vi "generateWaveform.vi"(8 "error in (no error)":errorcluster, 11 "GuassianNoiseWave in":refnum<class "GuassianNoiseWave.lvclass">) -> (0 "error out":errorcluster, 2 "signal out":waveform(dbl), 3 "GuassianNoiseWave out":refnum<class "GuassianNoiseWave.lvclass">)   [LabVIEW 2015, in "GuassianNoiseWave.lvclass"]
uses:
  GuassianNoiseWave.lvclass
  GuassianNoiseWave.lvclass/GuassianNoiseWave.ctl
  <vilib>/Waveform/WDTOps.llb/WDT Append Waveforms DBL.vi
  <vilib>/measure/NI_MABase.lvlib
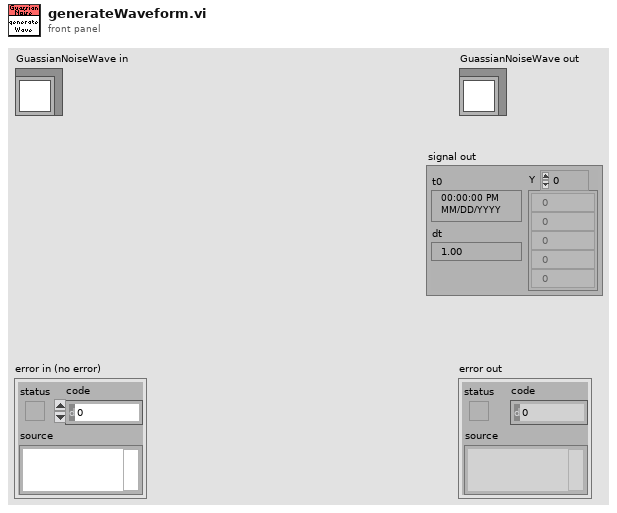
[diagram p1: front panel]
types:
  T1 = typedef "FAMTTypedefs.lvlib/Iterations.ctl" = i32
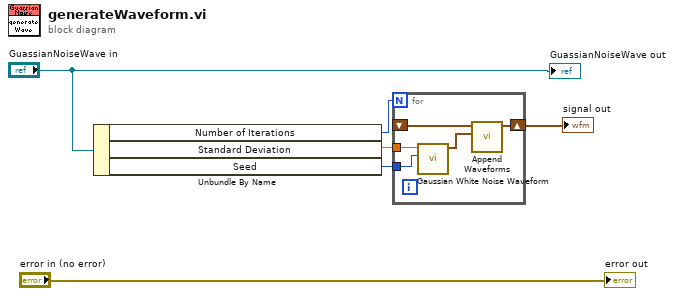
[diagram p0: block diagram]
diagram:
  n1 = Unbundle By Name("GuassianNoiseWave in") -> ("Number of Iterations"=w4:T1, "Standard Deviation"=w6:dbl, "Seed"=w5:i32)
  n2 = for {
    N: w4 -> [_]
    tunnel: w6 -> [w11]
    tunnel: w5 -> [w10]
    shift-right: [w8] -> w2
    shift-left: _ -> [w7]
    n3 = call <vilib>:"Gaussian White Noise Waveform.vi"("seed"=w10, "standard deviation"=w11) -> ("signal out"=w9:waveform(dbl))  [unwired: 8 in, 1 out]
    n4 = call-poly <vilib>:"Append Waveforms.vi"("waveform B"=w9, "waveform A"=w7) -> ("waveform out"=w8:waveform(dbl))  [unwired: 8 in, 1 out]
  }
  "signal out" <- w2
  "error out" <- "error in (no error)"
  "GuassianNoiseWave out" <- "GuassianNoiseWave in"
